vi "chart set series gap.vi"(8 "error in (no error)":errorcluster, 10 "gap":u16, 11 "chart":u32) -> (0 "error out":errorcluster)   [LabVIEW 8.6]
doc: "void chart_set_series_gap(lxw_chart chart, uint16_t gap);"
uses:
  pending_lvxlsxwriter/xlsxwriter.dll
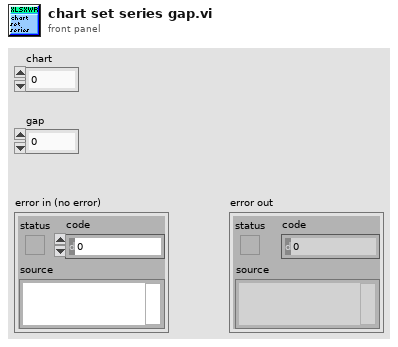
[diagram p1: front panel]
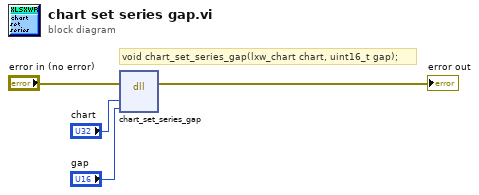
[diagram p0: block diagram]
diagram:
  # "void chart_set_series_gap(lxw_chart chart, uint16_t gap);"
  n1 = dll-call lib="C:/Users/WDAGUtilityAccount/Desktop/pending_lvxlsxwriter/xlsxwriter.*" fn="chart_set_series_gap"(error in="error in (no error)", "chart"="chart", "gap"="gap") -> (error out=→"error out":errorcluster)  [unwired: 5 in, 1 out]
